vi "Get Frame.vi"(8 "error in (no error)":errorcluster, 10 "timeout":i32=10000, 11 "VideoScanCamera in":refnum<class "VideoScanDeviceLibrary.lvclass">) -> (0 "error out":errorcluster, 1 "error?":bool, 2 "Frame":u16[][](array[numeric]), 3 "VideoScanCamera out":refnum<class "VideoScanDeviceLibrary.lvclass">)   [LabVIEW 2014, in "VideoScanDeviceLibrary.lvclass"]
uses:
  VideoScanDeviceLibrary.lvclass
  <vilib>/Utility/error.llb/DialogType.ctl
  VideoScanDeviceLibrary.lvclass/VideoScanDeviceLibrary.ctl
  <vilib>/MediaMongrels Ltd/WebSockets/WebSockets/WebSockets.lvlib
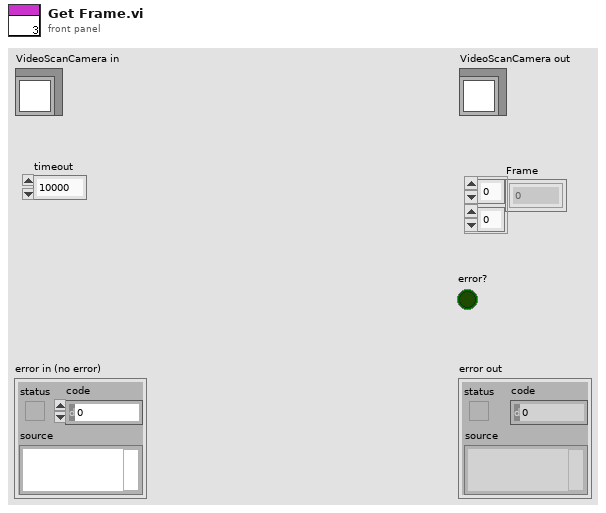
[diagram p1: front panel]
types:
  T1 = typedef "DialogType.ctl" = u16
  T2 = typedef "WebSockets.lvlib/Opcodes.ctl" = u8
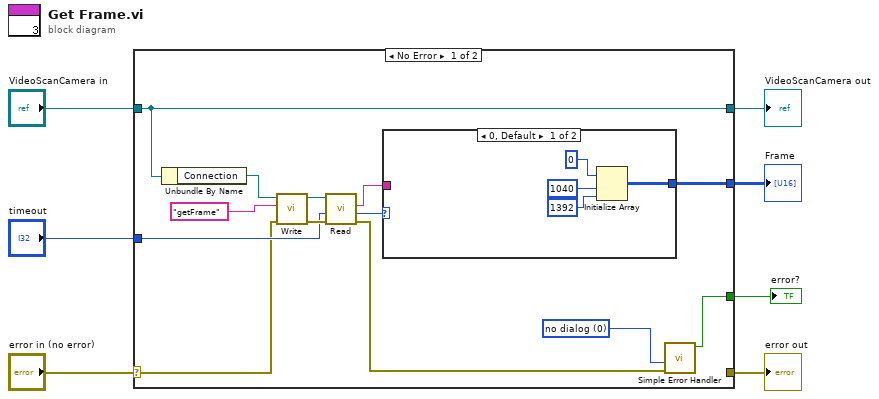
[diagram p0: block diagram]
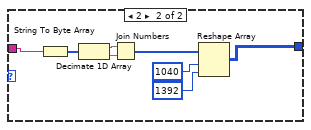
[diagram p2: hidden frame]
diagram:
  n1 = case shown="No Error" "error in (no error)" {
    selector: "error in (no error)" -> [w12 w34]
    tunnel: [_ w34] -> w6
    tunnel: [w14 w33] -> w4
    tunnel: "VideoScanCamera in" -> [w14 w33]
    tunnel: "timeout" -> [w17 _]
    tunnel: [w11 _] -> w2
    tunnel: [w9 _] -> w1
    frame No Error {
      w10 = T1 0 items=["no dialog", "OK message", "continue or stop message", "OK message + warnings", "continue/stop + warnings"] ("type of dialog (OK msg:1)")
      n2 = Unbundle By Name(w14) -> ("Connection"=w13:refnum<k5>)
      n3 = call <vilib>:"Write.vi"("error in (no error)"=w12, "Data"="getFrame", "WebSocket Connection in"=w13) -> ("error out"=w19:errorcluster, "WebSocket Connection out"=w18:refnum<k5>)  [unwired: 7 in]
      n4 = call <vilib>:"Read.vi"("error in (no error)"=w19, "timeout ms (5000)"=w17, "WebSocket Connection in"=w18) -> ("error out"=w8:errorcluster, "Opcode"=w16:T2, "Data"=w15:string)  [unwired: 4 in, 2 out]
      n5 = case shown="0, Default" w16 {
        tunnel: w15 -> [_ w26]
        tunnel: [w21 w25] -> w11
        frame 0, Default {
          n6 = Initialize Array(u16 0 ("element"), 1040 ("dimension size"), 1392 ("dimension size")) -> (w21:u16[][])
        }
        frame 2 {
          n7 = String To Byte Array(string=w26) -> (unsigned byte array=w32:u8[])
          n8 = Decimate 1D Array(w32) -> (w31:u8[], w30:u8[])
          n9 = Join Numbers(hi=w31, lo=w30) -> ((hi.lo)=w29:u16[])
          n10 = Reshape Array(w29, 1040 ("dimension size"), 1392 ("dimension size")) -> (w25:u16[][])
        }
      }
      n11 = call <vilib>:"Simple Error Handler.vi"("type of dialog (OK msg:1)"=w10, "error in (no error)"=w8) -> ("error?"=w9:bool)  [unwired: 3 in, 4 out]
    }
    frame Error {
    }
  }
  "error out" <- w6
  "VideoScanCamera out" <- w4
  "Frame" <- w2
  "error?" <- w1
